vi "DB Module.vi"(8 "error in":errorcluster) -> (0 "error out":errorcluster)   [LabVIEW 2025, in "Config Database.lvlib"]
doc: "This is the top level module for the config database (a free running module of the ATM simulator). \n\nDeveloper must create API for the DB module to return values to the controller. In the controller, replace this VI with the appropriate API. Use the UIs ( x 3) and controller as examples of how the API is to be built.\n\nIt is closed using a user event. It communicates with the other modules using a\nqueue based API which has comms modules that can be swapped if required."
uses:
  Config Database.lvlib
  Private Controls/DB Data.ctl
  Private Controls/Module Data Cluster.ctl
  Private Controls/Module Action.ctl
  Error Handler/Error Handler.lvlib
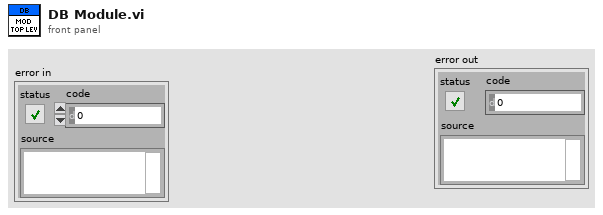
[diagram p1: front panel]
types:
  T1 = typedef "Config Database.lvlib/DB Data.ctl" = cluster{"Account":dbl[], "First Name":string[], "Last Name":string[], "Balance":dbl[]}
  T2 = typedef "Config Database.lvlib/Module Data Cluster.ctl" = cluster{"Data":variant, "Action":T3}
  T3 = typedef "Config Database.lvlib/Module Action.ctl" = enum16{"Get balance", "Find Account", "Update balance", "Error", "Exit", "Init"}
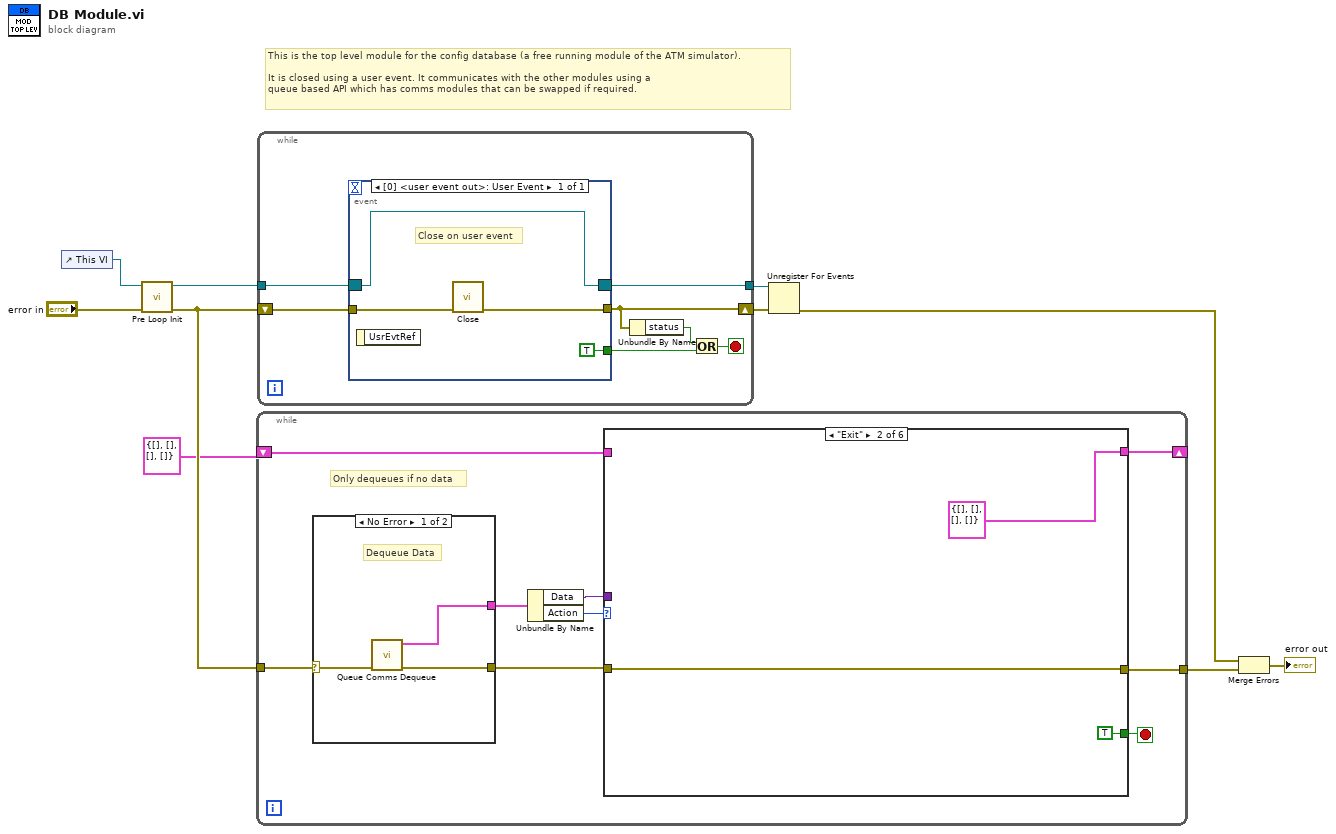
[diagram p0: block diagram]
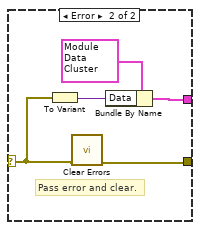
[diagram p2: hidden frame]
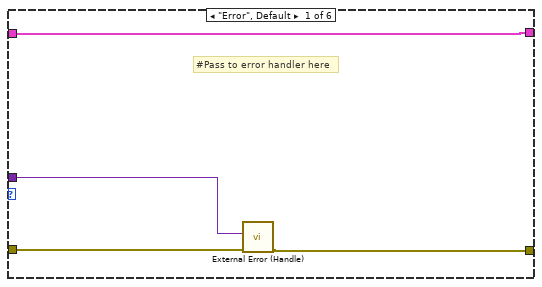
[diagram p3: hidden frame]
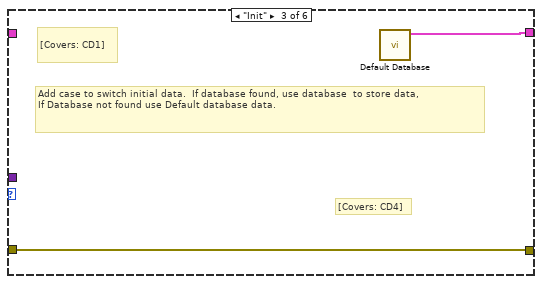
[diagram p4: hidden frame]
diagram:
  # "This is the top level module for the config database (a free running module of the ATM simulator). \n\nIt is closed using a user event. It communicates with the other modules using a\nqueue based API which has comms modules that can be swapped if required."
  n1 = control-ref of="This VI"() -> (w10:refnum<vi>)
  n2 = call "Pre Loop Init.vi"("error in"="error in", "Ref In"=w10) -> ("error out"=w5:errorcluster, "Event Registration Refnum"=w8:refnum<event-registration>)  [unwired: 8 in]
  n3 = while {
    tunnel: w5 -> [w18]
    tunnel: [w13] -> w3
    shift-right: [w12] -> _
    shift-left: T1 {"Account"=[], "First Name"=[], "Last Name"=[], "Balance"=[]} ("DB") -> [w11]
    stop <- w19 stop-if-true
    # "Only dequeues if no data"
    n4 = case shown="No Error" w18 {
      selector: w18 -> [w21 w24]
      tunnel: [w22 w23] -> w16
      tunnel: [w20 w25] -> w17
      frame No Error {
        # "Dequeue Data"
        n5 = call "Queue Comms Dequeue.vi"("error in"=w21) -> ("error out"=w22:errorcluster, "Data Out"=w20:T2)  [unwired: 9 in]
      }
      frame Error {
        # "Pass error and clear."
        n6 = To Variant(anything=w24) -> (Variant=w26:variant)
        n7 = call <vilib>:"Clear Errors.vi"("error in (no error)"=w24) -> ("error out"=w23:errorcluster)  [unwired: 5 in, 1 out]
        n8 = Bundle By Name(cluster=T2 {"Data"=variant, "Action"=enum."Error"} ("Cluster"), "Data"=w26) -> (w25:T2)
      }
    }
    n9 = Unbundle By Name(w17) -> ("Data"=w14:variant, "Action"=w15:T3)
    n10 = case shown="\"Exit\"" w15 {
      tunnel: [_ TRUE _ _ _ _] -> w19
      tunnel: w16 -> [w31 w33 w36 w38 w40 w42]
      tunnel: w14 -> [w29 _ _ _ _ _]
      tunnel: [w30 w33 w36 w38 w40 w42] -> w13
      tunnel: [w28 T1 {"Account"=[], "First Name"=[], "Last Name"=[], "Balance"=[]} ("DB") w35 w37 w39 w41] -> w12
      tunnel: w11 -> [w28 _ _ w37 w39 w41]
      frame "Error", Default {
        # "#Pass to error handler here"
        n11 = call "External Error (Handle).vi"("error in"=w31, "Data"=w29) -> ("error out"=w30:errorcluster)  [unwired: 9 in]
      }
      frame "Exit" {
      }
      frame "Init" {
        # "[Covers: CD4]"
        # "Add case to switch initial data.  If database found, use database  to store data, \nIf Database not found use Default database data."
        # "[Covers: CD1]"
        n12 = call "Default Database.vi"() -> ("DB"=w35:T1)  [unwired: 10 in, 1 out]
      }
      frame "Find Account" {
        # "Create API to send value to controller"
        # "[Covers: CD5]"
        # "add code here to launch the record \nUser Interface.\n\nUsed to find Account Number \n[Covers: CD3]"
      }
      frame "Update balance" {
        # "Create API to send value to controller"
        # "[Covers: CD2]"
        # "[Covers: CD2A]"
        # "Develop method to update balance"
      }
      frame "Get balance" {
        # "Create API to send value to controller"
        # "[Covers: CD2]"
        # "Method to get balance"
      }
    }
  }
  n13 = while {
    shift-right: [w46] -> w7
    shift-left: w5 -> [w49]
    tunnel: w8 -> [w44]
    tunnel: [w43] -> w6
    stop <- w47 stop-if-true
    n14 = event shown="[0] <user event out>: User Event" {
      selector: w44 -> [w53]
      dyn-events: [w53] -> w43
      timeout: _ -> [_]
      tunnel: w49 -> [w52]
      tunnel: [w51] -> w46
      tunnel: [TRUE ("stop")] -> w48
      event User Event {
        # "Close on user event"
        n15 = event-data() -> ()  [unwired: 1 in, 1 out]
        n16 = call "Close.vi"("error in"=w52) -> ("error out"=w51:errorcluster)  [unwired: 10 in]
      }
    }
    n17 = Unbundle By Name(w46) -> ("status"=w45:bool)
    n18 = Or(x=w45, y=w48) -> (x .or. y?=w47:bool)
  }
  n19 = Unregister For Events(event registration refnum=w6, error in=w7) -> (error out=w2:errorcluster)
  n20 = Merge Errors(w2, w3) -> (→"error out":errorcluster)
